vi "ExpEval_CheckMatchingParenthesis.vi"(11 "expression in":string) -> (2 "match":bool, 3 "expression out":string)   [LabVIEW 2017, in "ExpressionEvaluator.lvlib"]
uses:
  <vilib>/addons/InsightCM/Utilities/ExpressionEvaluator/ExpressionEvaluator.lvlib
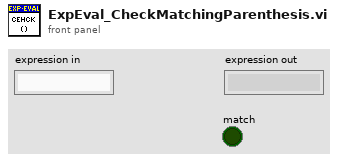
[diagram p1: front panel]
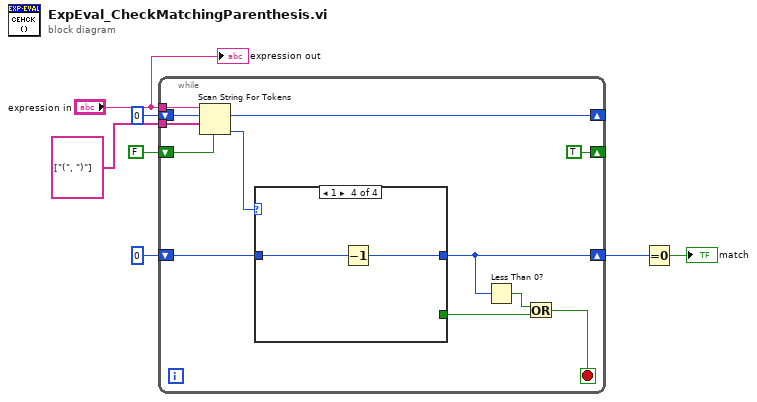
[diagram p0: block diagram]
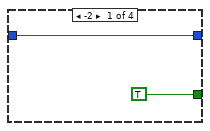
[diagram p2: hidden frame]
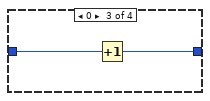
[diagram p4: hidden frame]
diagram:
  n1 = while {
    tunnel: "expression in" -> [w19]
    shift-right: [TRUE] -> _
    shift-left: FALSE -> [w18]
    tunnel: string[] ["(", ")"] -> [w16]
    shift-right: [w15] -> _
    shift-left: 0 ("offset past token") -> [w14]
    shift-right: [w9] -> w3
    shift-left: 0 ("offset past token") -> [w10]
    stop <- w11 stop-if-true
    n2 = Scan String For Tokens(4:w18, 7:w16, 8:w14, 9:w19) -> (0:w13:i32, 2:w15:i32)  [unwired: 2 in, 2 out]
    n3 = case shown="1" w13 {
      tunnel: [TRUE _ _ _] -> w12
      tunnel: [w20 w22 w23 w25] -> w9
      tunnel: w10 -> [w20 w22 w24 w26]
      frame -2 {
      }
      frame Default {
      }
      frame 0 {
        n4 = Increment(x=w24) -> (x+1=w23:i32)
      }
      frame 1 {
        n5 = Decrement(x=w26) -> (x-1=w25:i32)
      }
    }
    n6 = Less Than 0?(x=w9) -> (x < 0?=w8:bool)
    n7 = Or(x=w8, y=w12) -> (x .or. y?=w11:bool)
  }
  n8 = Equal To 0?(x=w3) -> (x = 0?=→"match":bool)
  "expression out" <- "expression in"
